vi "Cross-Talk, Calculate Current.vi"(7 "Waveform In":waveform(dbl), 8 "error in":errorcluster, 10 "Resistance (ohms)":dbl=nan format="%.1f") -> (0 "error out":errorcluster, 3 "Amplitude (uA)":dbl)   [LabVIEW 2010]
uses:
  <vilib>/measure/madcrms.llb/Basic Averaged DC-RMS for 1 Chan.vi
  <vilib>/measure/NI_MAPro.lvlib
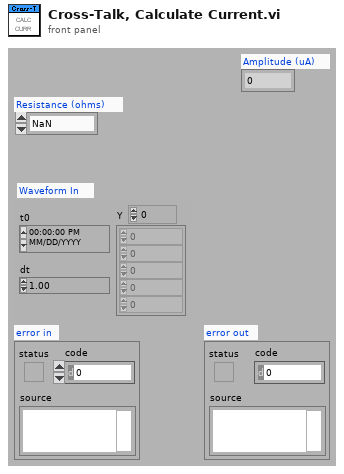
[diagram p1: front panel]
types:
  T1 = enum16{"Rectangular (none)", "Hanning", "Low side lobe"}
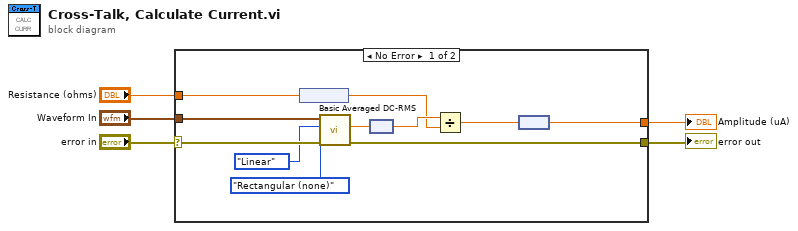
[diagram p0: block diagram]
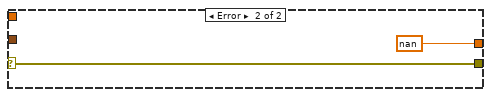
[diagram p2: hidden frame]
diagram:
  n1 = case shown="No Error" "error in" {
    selector: "error in" -> [w12 w17]
    tunnel: "Waveform In" -> [w15 _]
    tunnel: "Resistance (ohms)" -> [w16 _]
    tunnel: [w14 nan ("Value")] -> w4
    tunnel: [w13 w17] -> w3
    frame No Error {
      n2 = node(w16) -> (w8:dbl[unit])
      n3 = call-poly <vilib>:"Basic Averaged DC-RMS.vi"("error in (no error)"=w12, "window"=T1."Rectangular (none)", "averaging type"=enum16{"Linear", "Exponential"}."Linear", "signal in"=w15) -> ("error out"=w13:errorcluster, "RMS value"=w7:dbl)  [unwired: 4 in, 2 out]
      n4 = node(w7) -> (w11:dbl[unit])
      n5 = Divide(x=w11, y=w8) -> (x/y=w6:dbl[unit])
      n6 = node(w6) -> (w14:dbl)
    }
    frame Error {
    }
  }
  "Amplitude (uA)" <- w4
  "error out" <- w3
